vi "Receive Write Single Bit Response.vi"(8 "error in (no error)":errorcluster, 11 "Port Selection Info":T1={"Port Name"="", "Amplifier Num"=1, "Baud Rate"=38400, "Char Formation"=enum."0"} {"Baud Rate" items=["38400"=38400, "19200"=19200, "9600"=9600, "115200"=0]; "Amplifier Num" max=31}) -> (0 "error out":errorcluster, 1 "ON/OFF":bool, 2 "Address":u16=4102 format="%.0x", 3 "Port Selection Info Out":T1={"Port Name"="", "Amplifier Num"=1, "Baud Rate"=38400, "Char Formation"=enum."0"} {"Baud Rate" items=["38400"=38400, "19200"=19200, "9600"=9600, "115200"=0]; "Amplifier Num" max=31}, 4 "CRC Match":bool, 5 "FC":u8=5, 7 "Bank":u8)   [LabVIEW 2014, in "ALPHA5 RS485.lvlib"]
uses:
  ALPHA5 RS485.lvlib
  typedefs/Port Selection Info.ctl
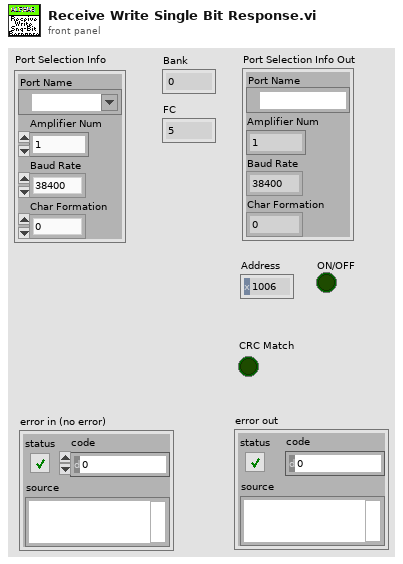
[diagram p1: front panel]
types:
  T1 = typedef "ALPHA5 RS485.lvlib/Port Selection Info.ctl" = cluster{"Port Name":refnum<visa-resource-name>, "Amplifier Num":u8, "Baud Rate":u32, "Char Formation":enum16{"0", "1", "2", "3", "4", "5"}}
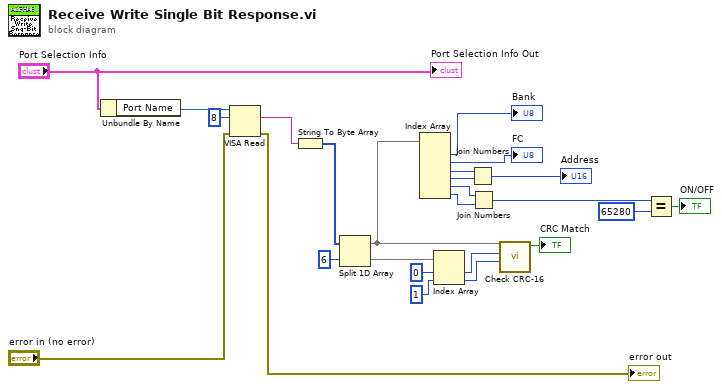
[diagram p0: block diagram]
diagram:
  n1 = Unbundle By Name("Port Selection Info") -> ("Port Name"=w24:refnum<visa-resource-name>)
  n2 = VISA Read(VISA resource name=w24, byte count=u32 8, error in (no error)="error in (no error)") -> (read buffer=w21:string, error out=→"error out":errorcluster)  [unwired: 2 out]
  n3 = String To Byte Array(string=w21) -> (unsigned byte array=w13:u8[])
  n4 = Split 1D Array(array=w13, index=6) -> (first subarray=w6:u8[], second subarray=w8:u8[])
  n5 = Index Array(array=w6) -> (element #1=→"Bank":u8, element #2=→"FC":u8, element #3=w18:u8, element #4=w17:u8, element #5=w15:u8, element #6=w14:u8)  [unwired: 6 in]
  n6 = Index Array(array=w8, index #1=0 ("index"), index #2=1 ("index")) -> (element #1=w7:u8, element #2=w9:u8)
  n7 = Join Numbers(hi=w18, lo=w17) -> ((hi.lo)=→"Address":u16)
  n8 = Join Numbers(hi=w15, lo=w14) -> ((hi.lo)=w3:u16)
  n9 = call "Check CRC-16.vi"("CRC-16-H"=w9, "CRC-16-L"=w7, "Data In"=w6) -> ("Check Result"=→"CRC Match":bool)  [unwired: 7 in, 1 out]
  n10 = Equal?(x=w3, y=u16 65280) -> (x = y?=→"ON/OFF":bool)
  "Port Selection Info Out" <- "Port Selection Info"
